vi "Set WLAN Type.vi"(8 "error in (no error)":errorcluster, 10 "WLAN Type":T1, 11 "niDTS WLAN Dut in":refnum<class "niDTS WLAN Dut.lvclass">) -> (0 "error out":errorcluster, 3 "niDTS WLAN Dut out":refnum<class "niDTS WLAN Dut.lvclass">)   [LabVIEW 2015, in "niDTS WLAN.lvlib" / "niDTS WLAN Dut.lvclass"]
doc: "Sets the Standard, Rate, and Streams comensurate with the input. \n\nCallbacks: Update Payload Length"
uses:
  niDTS WLAN Dut.lvclass
  Includes/niDTS WLAN INC Type.ctl
  niDTS WLAN Dut.lvclass/niDTS WLAN Dut.ctl
  niDTS WLAN.lvlib
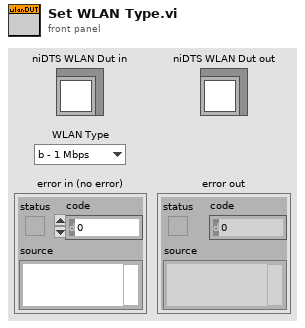
[diagram p1: front panel]
types:
  T1 = typedef "niDTS WLAN.lvlib/niDTS WLAN INC Type.ctl" = enum16{"b - 1 Mbps", "b - 2 Mbps", "b - 5.5 Mbps", "b - 11 Mbps", "ag - 6 Mbps", "ag - 9 Mbps", "ag - 12 Mbps", "ag - 18 Mbps", "ag - 24 Mbps", "ag - 36 Mbps", "ag - 48 Mbps", "ag - 54 Mbps", "n - MCS0", "n - MCS1", "n - MCS2", "n - MCS3", "n - MCS4", "n - MCS5", "n - MCS6", "n - MCS7", "n - MCS8", "n - MCS9", "n - MCS10", "n - MCS11", "n - MCS12", "n - MCS13", "n - MCS14", "n - MCS15", "n - MCS16", "n - MCS17", "n - MCS18", "n - MCS19", "n - MCS20", "n - MCS21", "n - MCS22", "n - MCS23", "n - MCS24", "n - MCS25", "n - MCS26", "n - MCS27", "n - MCS28", "n - MCS29", "n - MCS30", "n - MCS31", "ac - MCS0 -1", "ac - MCS1 -1", "ac - MCS2 -1", "ac - MCS3 -1", "ac - MCS4 -1", "ac - MCS5 -1", "ac - MCS6 -1", "ac - MCS7 -1", "ac - MCS8 -1", "ac - MCS9 -1", "ac - MCS0 -2", "ac - MCS1 -2", "ac - MCS2 -2", "ac - MCS3 -2", "ac - MCS4 -2", "ac - MCS5 -2", "ac - MCS6 -2", "ac - MCS7 -2", "ac - MCS8 -2", "ac - MCS9 -2", "ac - MCS0 -3", "ac - MCS1 -3", "ac - MCS2 -3", "ac - MCS3 -3", "ac - MCS4 -3", "ac - MCS5 -3", "ac - MCS6 -3", "ac - MCS7 -3", "ac - MCS8 -3", "ac - MCS9 -3", "ac - MCS0 -4", "ac - MCS1 -4", "ac - MCS2 -4", "ac - MCS3 -4", "ac - MCS4 -4", "ac - MCS5 -4", "ac - MCS6 -4", "ac - MCS7 -4", "ac - MCS8 -4", "ac - MCS9 -4"}
  T2 = typedef "niDTS WLAN.lvlib/niDTS WLAN INC Standard.ctl" = enum16{"802.11 b DSSS", "802.11 a/g OFDM", "802.11 n HT", "802.11 ac VHT"}
  T3 = typedef "niDTS WLAN.lvlib/niDTS WLAN INC DSSS Data Rate.ctl" = enum16{"1", "2", "5.5", "11"}
  T4 = typedef "niDTS WLAN.lvlib/niDTS WLAN INC OFDM Data Rate.ctl" = enum16{"6", "9", "12", "18", "24", "36", "48", "54"}
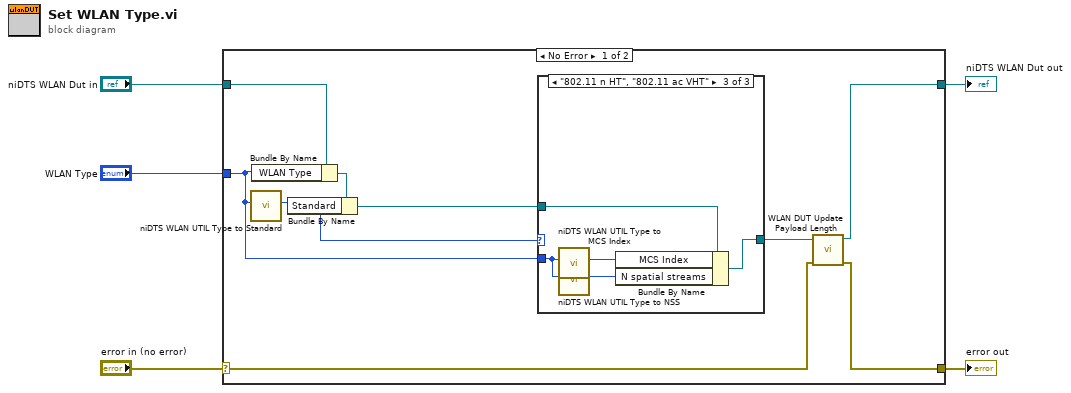
[diagram p0: block diagram]
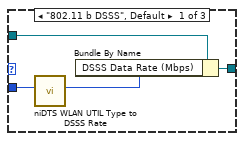
[diagram p2: hidden frame]
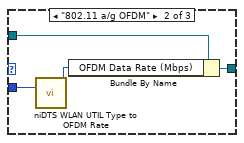
[diagram p3: hidden frame]
diagram:
  n1 = case shown="No Error" "error in (no error)" {
    selector: "error in (no error)" -> [w8 w28]
    tunnel: [w7 w28] -> w4
    tunnel: [w6 w29] -> w2
    tunnel: "niDTS WLAN Dut in" -> [w14 w29]
    tunnel: "WLAN Type" -> [w11 _]
    frame No Error {
      n2 = call "niDTS WLAN UTIL Type to Standard.vi"("WLAN Type"=w11) -> ("Standard"=w10:T2)  [unwired: 10 in]
      n3 = Bundle By Name(cluster=w14, "WLAN Type"=w11) -> (w13:refnum<class "niDTS WLAN Dut.lvclass">)
      n4 = Bundle By Name(cluster=w13, "Standard"=w10) -> (w12:refnum<class "niDTS WLAN Dut.lvclass">)
      n5 = case shown="\"802.11 n HT\", \"802.11 ac VHT\"" w10 {
        tunnel: w12 -> [w17 w22 w27]
        tunnel: w11 -> [w18 w20 w24]
        tunnel: [w15 w21 w26] -> w9
        frame "802.11 b DSSS", Default {
          n6 = call "niDTS WLAN UTIL Type to DSSS Rate.vi"("WLAN Type"=w18) -> ("DSSS Data Rate (Mbps)"=w16:T3)  [unwired: 10 in]
          n7 = Bundle By Name(cluster=w17, "DSSS Data Rate (Mbps)"=w16) -> (w15:refnum<class "niDTS WLAN Dut.lvclass">)
        }
        frame "802.11 a/g OFDM" {
          n8 = call "niDTS WLAN UTIL Type to OFDM Rate.vi"("WLAN Type"=w20) -> ("OFDM Data Rate (Mbps)"=w19:T4)  [unwired: 10 in]
          n9 = Bundle By Name(cluster=w22, "OFDM Data Rate (Mbps)"=w19) -> (w21:refnum<class "niDTS WLAN Dut.lvclass">)
        }
        frame "802.11 n HT", "802.11 ac VHT" {
          n10 = call "niDTS WLAN UTIL Type to MCS Index.vi"("WLAN Type"=w24) -> ("MCS Index"=w25:i32)  [unwired: 10 in]
          n11 = call "niDTS WLAN UTIL Type to NSS.vi"("WLAN Type"=w24) -> ("NSS"=w23:i32)  [unwired: 10 in]
          n12 = Bundle By Name(cluster=w27, "MCS Index"=w25, "N spatial streams"=w23) -> (w26:refnum<class "niDTS WLAN Dut.lvclass">)
        }
      }
      n13 = call-dynamic "WLAN DUT Update Payload Length.vi"("error in (no error)"=w8, "niDTS WLAN DUT in"=w9) -> ("error out"=w7:errorcluster, "niDTS WLAN DUT out"=w6:refnum<class "niDTS WLAN Dut.lvclass">)  [unwired: 8 in]
    }
    frame Error {
    }
  }
  "error out" <- w4
  "niDTS WLAN Dut out" <- w2
